vi "Read Cycle Time (ms).vi"(8 "error in (no error)":errorcluster, 11 "Query in":refnum<class "Query.lvclass">) -> (0 "error out":errorcluster, 2 "Cycle Time (ms)":u32, 3 "Query out":refnum<class "Query.lvclass">)   [LabVIEW 2024, in "Query.lvclass"]
doc: "Query.lvclass:Read Cycle Time.vi\n\nThis VI is the accessor for the Cycle Time parameter for the Query class.\n\nInstrument Communication Module Version 1.0\nDecember, 2017 Original Code Consulting David Thomson\n www.originalcode.com"
uses:
  Query.lvclass
  Query.lvclass/Query.ctl
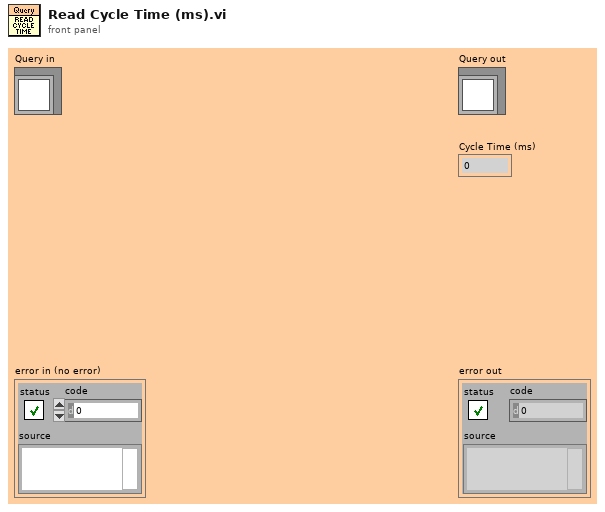
[diagram p1: front panel]
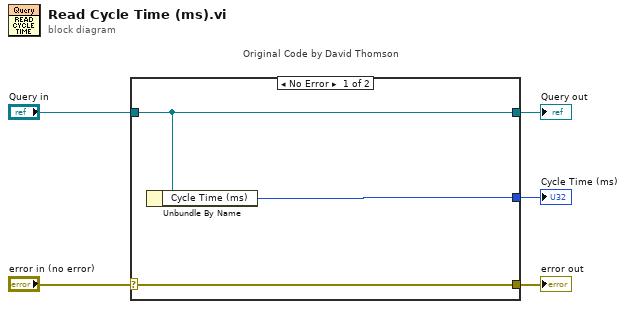
[diagram p0: block diagram]
diagram:
  n1 = case "Original Code by David Thomson" shown="No Error" "error in (no error)" {
    selector: "error in (no error)" -> [w8 w9]
    tunnel: [w8 w9] -> w4
    tunnel: [w7 w10] -> w2
    tunnel: "Query in" -> [w7 w10]
    tunnel: [w6 _] -> w1
    frame No Error {
      n2 = Unbundle By Name(w7) -> ("Cycle Time (ms)"=w6:u32)
    }
    frame Error {
    }
  }
  "error out" <- w4
  "Query out" <- w2
  "Cycle Time (ms)" <- w1
